vi "SelectRingMaker.vi"() -> ()   [LabVIEW 2013]
uses:
  <vilib>/regexp/Match Regular Expression.xnode
panel:
  in  "SelectRing":u16(ring) items=["臺北市", "新北市", "臺中市", "臺南市", "高雄市", "基隆市", "桃園縣", "新竹市", "新竹縣", "苗栗縣", "彰化縣", "雲林縣", "嘉義市", "嘉義縣", "屏東縣", "宜蘭縣", "花蓮縣", "臺東縣", "澎湖縣", "金門縣", "連江縣"]
  in  "SelectItemHtmlString":string="          <select name=\"menu1\" onChange=\"MM_jumpMenu('self',this,0)\">  <option value=\"Taipei_City.htm\">臺北市</option>  <option value=\"New_Taipei_City.htm\">新北市</option>  <option value=\"Taichung_City.htm\">臺中市</option>  <option value=\"Tainan_City.htm\">臺南市</option>  <option value=\"Kaohsiung_City.htm\">高雄市</option>  <option value=\"Keelung_City.htm\">基隆市</option>  <option value=\"Taoyuan_County.htm\">桃園縣</option>  <option value=\"Hsinchu_City.htm\">新竹市</option>  <option value=\"Hsinchu_County.htm\">新竹縣</option>  <option value=\"Miaoli_County.htm\">苗栗縣</option>  <option value=\"Changhua_County.htm\">彰化縣</option>  <option value=\"Nantou_County.htm\" selected=\"selected\">南投縣</option>  <option value=\"Yunlin_County.htm\">雲林縣</option>  <option value=\"Chiayi_City.htm\">嘉義市</option>  <option value=\"Chiayi_County.htm\">嘉義縣</option>  <option value=\"Pingtung_County.htm\">屏東縣</option>  <option value=\"Yilan_County.htm\">宜蘭縣</option>  <option value=\"Hualien_County.htm\">花蓮縣</option>  <option value=\"Taitung_County.htm\">臺東縣</option>  <option value=\"Penghu_County.htm\">澎湖縣</option>  <option value=\"Kinmen_County.htm\">金門縣</option>  <option value=\"Lienchiang_County.htm\">連江縣</option>          </select>\n"
  out "urlString":string[](array[string])
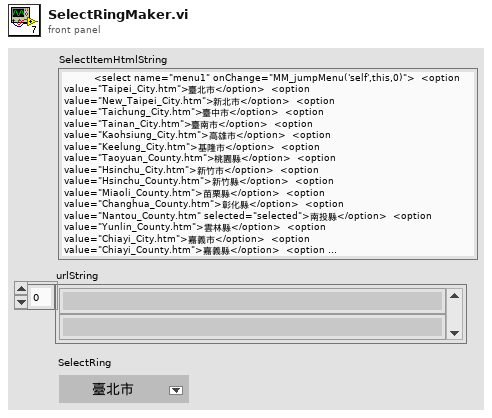
[diagram p1: front panel]
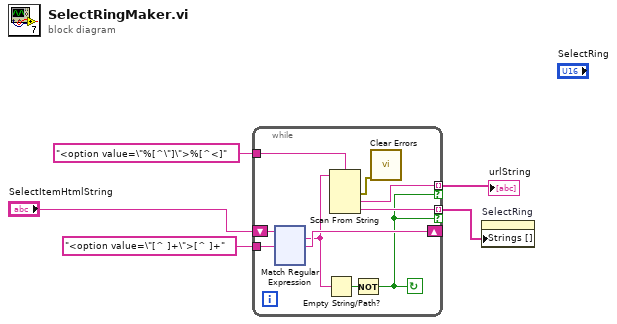
[diagram p0: block diagram]
diagram:
  n1 = while {
    tunnel: "<option value=\"[^ ]+\">[^ ]+" -> [w14]
    shift-right: [w13] -> _
    shift-left: "SelectItemHtmlString" -> [w15]
    tunnel: [w9] -> w3 mode=indexing if=w6
    tunnel: "<option value=\"%[^\"]\">%[^<]" -> [w10]
    tunnel: [w8] -> w1 mode=indexing if=w6
    stop <- w6 continue-if-true
    n2 = xnode "Match Regular Expression"("input string"=w15, "regular expression"=w14) -> ("whole match"=w11:string, "after match"=w13:string)  [unwired: 4 in, 3 out]
    n3 = Empty String/Path?(string/path=w11) -> (empty?=w12:bool)
    n4 = Scan From String(format string=w10, input string=w11) -> (error out=w7:errorcluster, output 1=w9:string, output 2=w8:string)  [unwired: 4 in, 2 out]
    n5 = Not(x=w12) -> (.not. x?=w6:bool)
    n6 = call <vilib>:"Clear Errors.vi"("error in (no error)"=w7) -> ()  [unwired: 6 in, 1 out]
  }
  "urlString" <- w3
  n7 = property on="SelectRing" class="Ring (strict)"("Strings []"=w1) -> ()  [unwired: 2 in, 2 out]
